vi "Run Test Method.vi"(8 "error in (no error)":errorcluster, 11 "LUnit Test Case In":refnum<class "LUnit Test Case.lvclass">) -> (0 "error out":errorcluster, 1 "Execution Time":dbl, 3 "LUnit Test Case Out":refnum<class "LUnit Test Case.lvclass">)   [LabVIEW 2020, in "LUnit Test Case.lvclass"]
uses:
  LUnit Test Case.lvclass
  LUnit Test Case.lvclass/LUnit Test Case.ctl
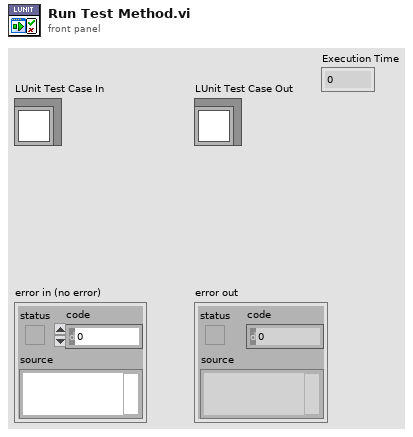
[diagram p1: front panel]
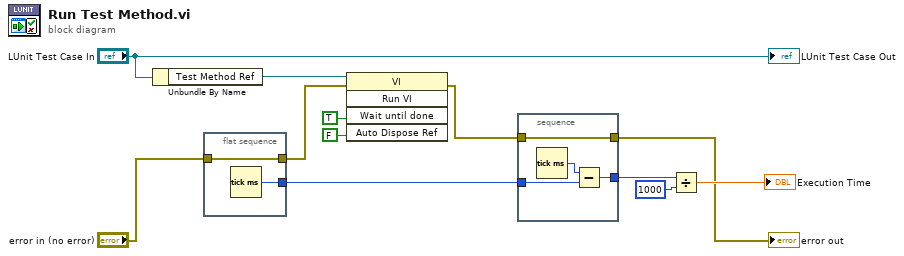
[diagram p0: block diagram]
diagram:
  n1 = Unbundle By Name("LUnit Test Case In") -> ("Test Method Ref"=w8:refnum<vi>)
  n2 = flat-sequence {
    tunnel: "error in (no error)" -> [w14]
    tunnel: [w14] -> w5
    tunnel: [w13] -> w3
    frame #0 {
      n3 = Tick Count (ms)() -> (millisecond timer value=w13:u32)
    }
  }
  n4 = invoke class="VI" method="Run VI"(reference=w8, error in=w5, "Wait until done"=TRUE ("Wait Until Done"), "Auto Dispose Ref"=FALSE ("Auto Dispose Reference")) -> (error out=w4:errorcluster)  [unwired: 1 in, 4 out]
  n5 = stacked-sequence {
    tunnel: [w16] -> w1
    tunnel: [w17] -> w2
    tunnel: w4 -> [w16]
    tunnel: w3 -> [w15]
    frame #0 {
      n6 = Tick Count (ms)() -> (millisecond timer value=w18:u32)
      n7 = Subtract(x=w18, y=w15) -> (x-y=w17:u32)
    }
  }
  "error out" <- w1
  n8 = Divide(x=w2, y=u32 1000) -> (x/y=→"Execution Time":dbl)
  "LUnit Test Case Out" <- "LUnit Test Case In"
